vi "Aprox Equal Zero.vi"(10 "maxV (fps)":dbl) -> (2 "Boolean":bool)   [LabVIEW 2018]
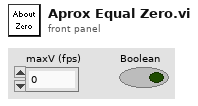
[diagram p1: front panel]
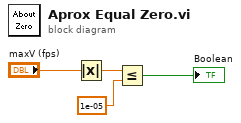
[diagram p0: block diagram]
diagram:
  n1 = Absolute Value(x="maxV (fps)") -> (abs(x)=w3:dbl)
  n2 = Less Or Equal?(x=w3, y=1e-05) -> (x <= y?=→"Boolean":bool)
